vi "Timescale_Check.vi"() -> (0 "Channel Indicies":i32[](array[numeric]))   [LabVIEW 2010]
uses:
  Globals/Meas_global.vi
  Globals/Dynamic_call_global.ph.vi
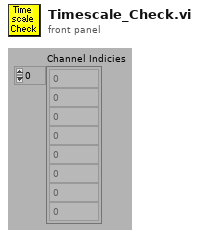
[diagram p1: front panel]
types:
  T1 = typedef "Analysis_type_cluster.ctl" = cluster{"Analysis type":T2, "Indicies":i32[], "Name":string, "Inst Array":T3, "Info index":i32}
  T2 = typedef "Analysis_type_Enum.ctl" = enum16{"Slow Response", "Fast Response", "Weighted Fast Response", "Fast FID", "Weighted Fast FID", "Cross Wire", "Weighted Cross Wire", "Weighted LDA"}
  T3 = typedef "Instrument_Array.ctl" = enum16{"PWA", "LDA", "Analogue"}
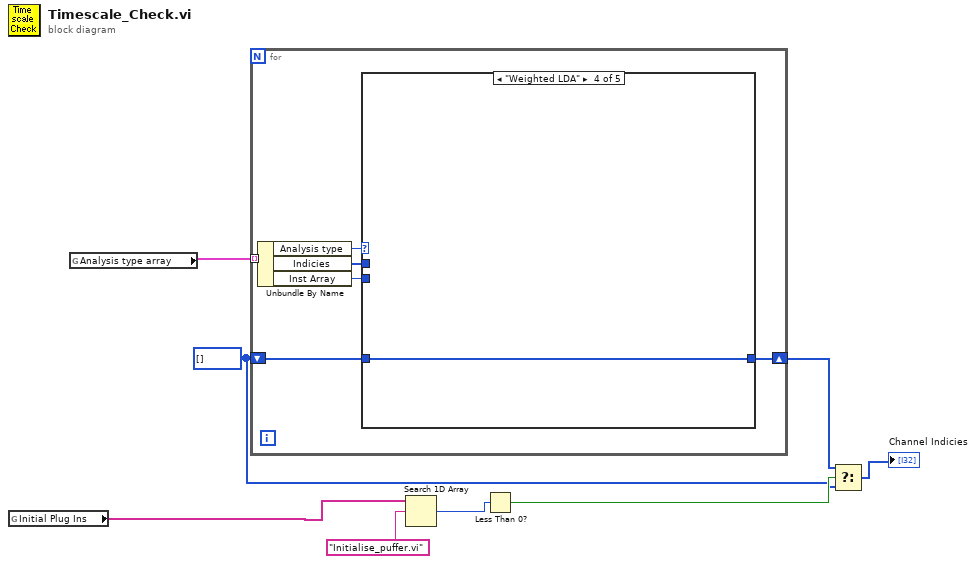
[diagram p0: block diagram]
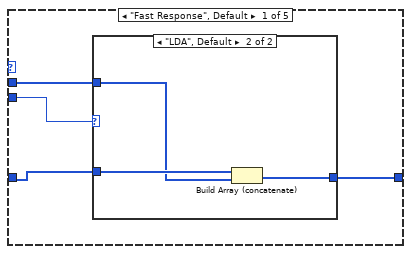
[diagram p2: hidden frame]
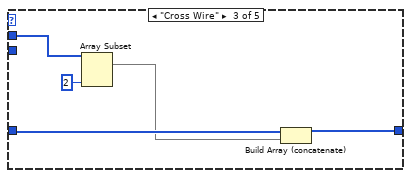
[diagram p5: hidden frame]
diagram:
  w3 = i32[] []
  n1 = global read "Dynamic_call_global.ph.vi" "Initial Plug Ins"() -> (w1:string[])
  n2 = global read "Meas_global.vi" "Analysis type array"() -> (w8:T1[])
  n3 = for {
    tunnel: w8 -> [w14] mode=indexing
    shift-right: [w11] -> w4
    shift-left: w3 -> [w12]
    n4 = Unbundle By Name(w14) -> ("Analysis type"=w13:T2, "Indicies"=w10:i32[], "Inst Array"=w9:T3)
    n5 = case shown="\"Weighted LDA\"" w13 {
      tunnel: w12 -> [w18 w23 w28 w29 w30]
      tunnel: [w16 w23 w27 w29 w30] -> w11
      tunnel: w10 -> [w17 _ w26 _ _]
      tunnel: w9 -> [w15 _ _ _ _]
      frame "Fast Response", Default {
        n6 = case shown="\"LDA\", Default" w15 {
          tunnel: w18 -> [w19 w22]
          tunnel: w17 -> [_ w21]
          tunnel: [w19 w20] -> w16
          frame "PWA" {
          }
          frame "LDA", Default {
            n7 = Build Array (concatenate)(w22, w21) -> (w20:i32[])
          }
        }
      }
      frame "Slow Response" {
      }
      frame "Cross Wire" {
        n8 = Array Subset(array=w26, length=2 ("Array Index")) -> (w25:i32[])  [unwired: 1 in]
        n9 = Build Array (concatenate)(w28, w25) -> (w27:i32[])
      }
      frame "Weighted LDA" {
      }
      frame "Weighted Fast Response" {
      }
    }
  }
  n10 = Search 1D Array(1D array=w1, element="Initialise_puffer.vi") -> (index of element=w6:i32)  [unwired: 1 out]
  n11 = Less Than 0?(x=w6) -> (x < 0?=w5:bool)
  n12 = Select(t=w4, s=w5, f=w3) -> (s? t:f=→"Channel Indicies":i32[])
